vi "Recoverty.vi"() -> ()   [LabVIEW 2011]
uses:
  <vilib>/Utility/file.llb/Write To Spreadsheet File (string).vi
panel:
  out "appended array":string[](array[string])
  out "error out":errorcluster
  in  "Name of File":string
  out "Elapsed Time (s)":dbl
  out "Read Value":dbl
  in  "resource name":refnum<visa-resource-name>
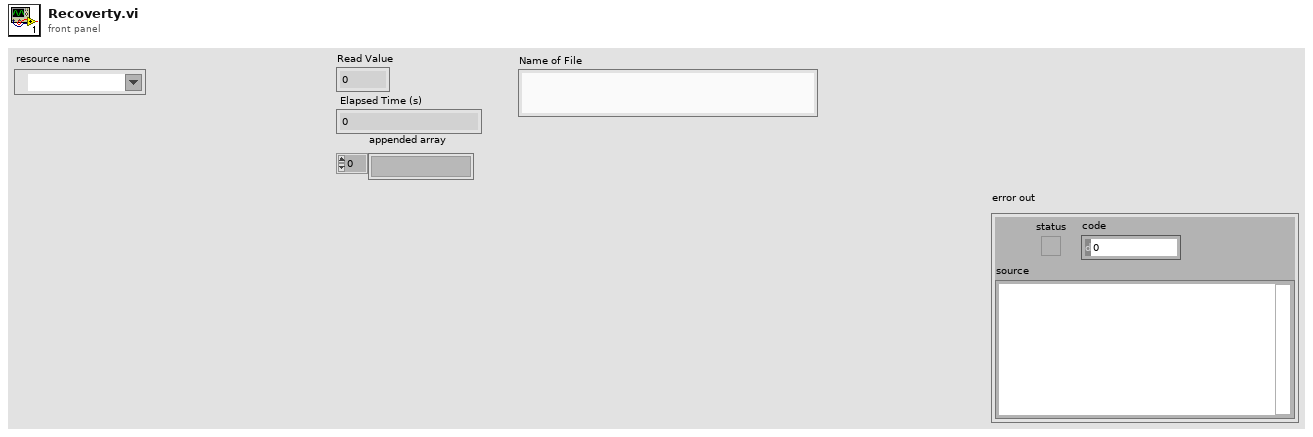
[diagram p1: front panel]
types:
  T1 = enum16{"open", "replace", "create", "open or create", "replace or create", "replace or create with confirmation"}
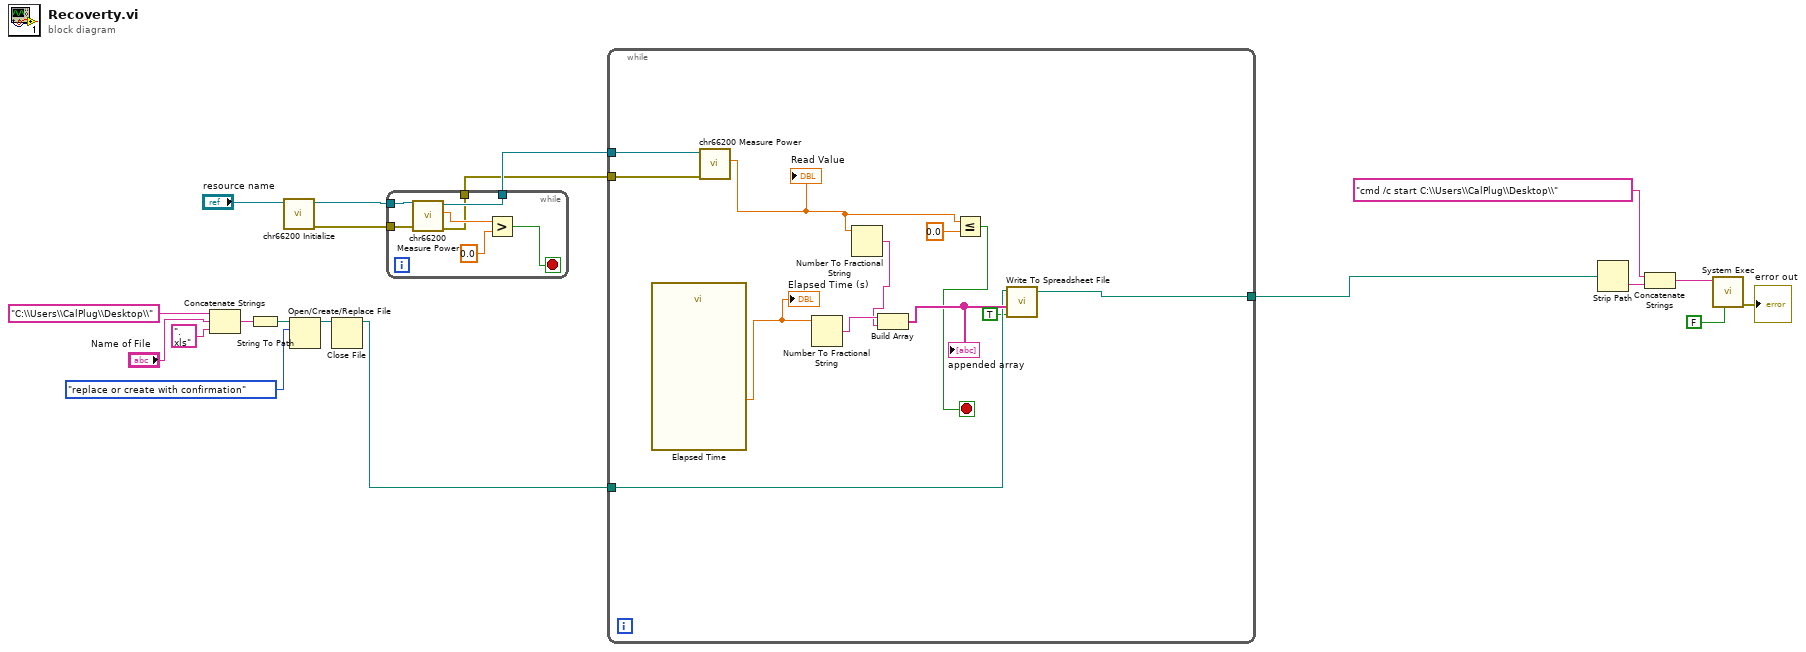
[diagram p0: block diagram]
diagram:
  n1 = Concatenate Strings("C:\\Users\\CalPlug\\Desktop\\" ("string"), "Name of File", ".xls" ("string")) -> (w15:string)
  n2 = String To Path(string=w15) -> (path=w16:path)
  n3 = call <instrlib>:"chr66200 Initialize.vi"("resource name"="resource name") -> ("error out"=w3:errorcluster, "instrument handle out"=w4:refnum<visa-resource-name>)  [unwired: 9 in]
  n4 = Open/Create/Replace File(file path (use dialog)=w16, operation (0:open)=T1."replace or create with confirmation") -> (refnum out=w14:refnum<file>)  [unwired: 4 in, 2 out]
  n5 = Close File(refnum=w14) -> (path=w13:path)  [unwired: 1 in, 1 out]
  n6 = while {
    tunnel: w4 -> [w24]
    tunnel: w3 -> [w23]
    tunnel: [w21] -> w2
    tunnel: [w20] -> w1
    stop <- w26 stop-if-true
    n7 = call <instrlib>:"chr66200 Measure Power.vi"("error in (no error)"=w23, "instrument handle"=w24) -> ("error out"=w20:errorcluster, "Read Value"=w22:dbl, "instrument handle out"=w21:refnum<visa-resource-name>)  [unwired: 7 in]
    n8 = Greater?(x=w22, y=0.0) -> (0:w26:bool)
  }
  n9 = while {
    tunnel: w13 -> [w36]
    tunnel: [w35] -> w7
    tunnel: w2 -> [w30]
    tunnel: w1 -> [w29]
    stop <- w31 stop-if-true
    n10 = call "Elapsed Time"() -> ("Elapsed Time (s)"=w27:dbl)  [unwired: 12 in, 7 out]
    "Elapsed Time (s)" <- w27
    n11 = call <instrlib>:"chr66200 Measure Power.vi"("error in (no error)"=w29, "instrument handle"=w30) -> ("Read Value"=w28:dbl)  [unwired: 7 in, 2 out]
    "Read Value" <- w28
    n12 = Number To Fractional String(number=w27) -> (F-format string=w38:string)  [unwired: 3 in]
    n13 = Number To Fractional String(number=w28) -> (F-format string=w34:string)  [unwired: 3 in]
    n14 = Build Array(w38, w34) -> (w37:string[])
    "appended array" <- w37
    n15 = Less Or Equal?(x=w28, y=0.0) -> (x <= y?=w31:bool)
    n16 = call-poly <vilib>:"Write To Spreadsheet File.vi"("append to file? (new file:F)"=TRUE, "1D data"=w37, "file path (dialog if empty)"=w36) -> ("new file path (Not A Path if cancelled)"=w35:path)  [unwired: 5 in]
  }
  n17 = Strip Path(path=w7) -> (name=w8:string)  [unwired: 1 out]
  n18 = Concatenate Strings("cmd /c start C:\\Users\\CalPlug\\Desktop\\" ("string"), w8) -> (w11:string)
  n19 = call <vilib>:"System Exec.vi"("run minimized? (F)"=FALSE, "command line"=w11) -> ("error out"=→"error out":errorcluster)  [unwired: 6 in, 3 out]
